vi "get Name.vi"(11 "Log in":refnum<class "Log.lvclass">) -> (3 "Name":string)   [LabVIEW 2020, in "Log.lvclass"]
uses:
  Log.lvclass
  Log.lvclass/Log.ctl
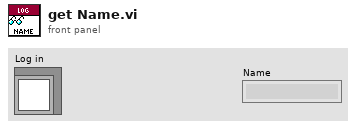
[diagram p1: front panel]
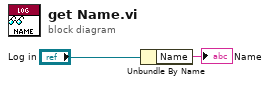
[diagram p0: block diagram]
diagram:
  n1 = Unbundle By Name("Log in") -> ("Name"=→"Name":string)
